vi "uc480_ImageSize.vi"() -> ()   [LabVIEW 2011]
uses:
  C:/Program Files/Thorlabs/Scientific Imaging/DCx Camera Support/Develop/DotNet/uc480DotNet.dll
  Develop/DotNet/uc480DotNet.dll
panel:
  out "Pos y":i32
  out "Pos x":i32
  out "AOI Height":i32
  out "AOI Width":i32
  in  "AOI - X Position":i32(slide)=33 min=0 max=0 step=2
  in  "AOI - Y Position":i32(slide)=33 min=0 max=0 step=2
  in  "AOI - Width":i32(slide)=16 min=16 max=1280 step=4 scale=16.0..1280.0
  in  "AOI - Height":i32(slide)=1 min=120 max=1024 step=2 scale=120.0..1024.0
  out "Image":picture
  in  "Camera ID":i32 min=0 max=255
  out "Serial Number":string
  out "Height":i32=8
  out "Width":i32=8
  out "Bits/Pixel":i32=8
  out "Error Out":errorcluster caption="error"
  in  "Exit Camera":bool
  in  "Init Camera":bool
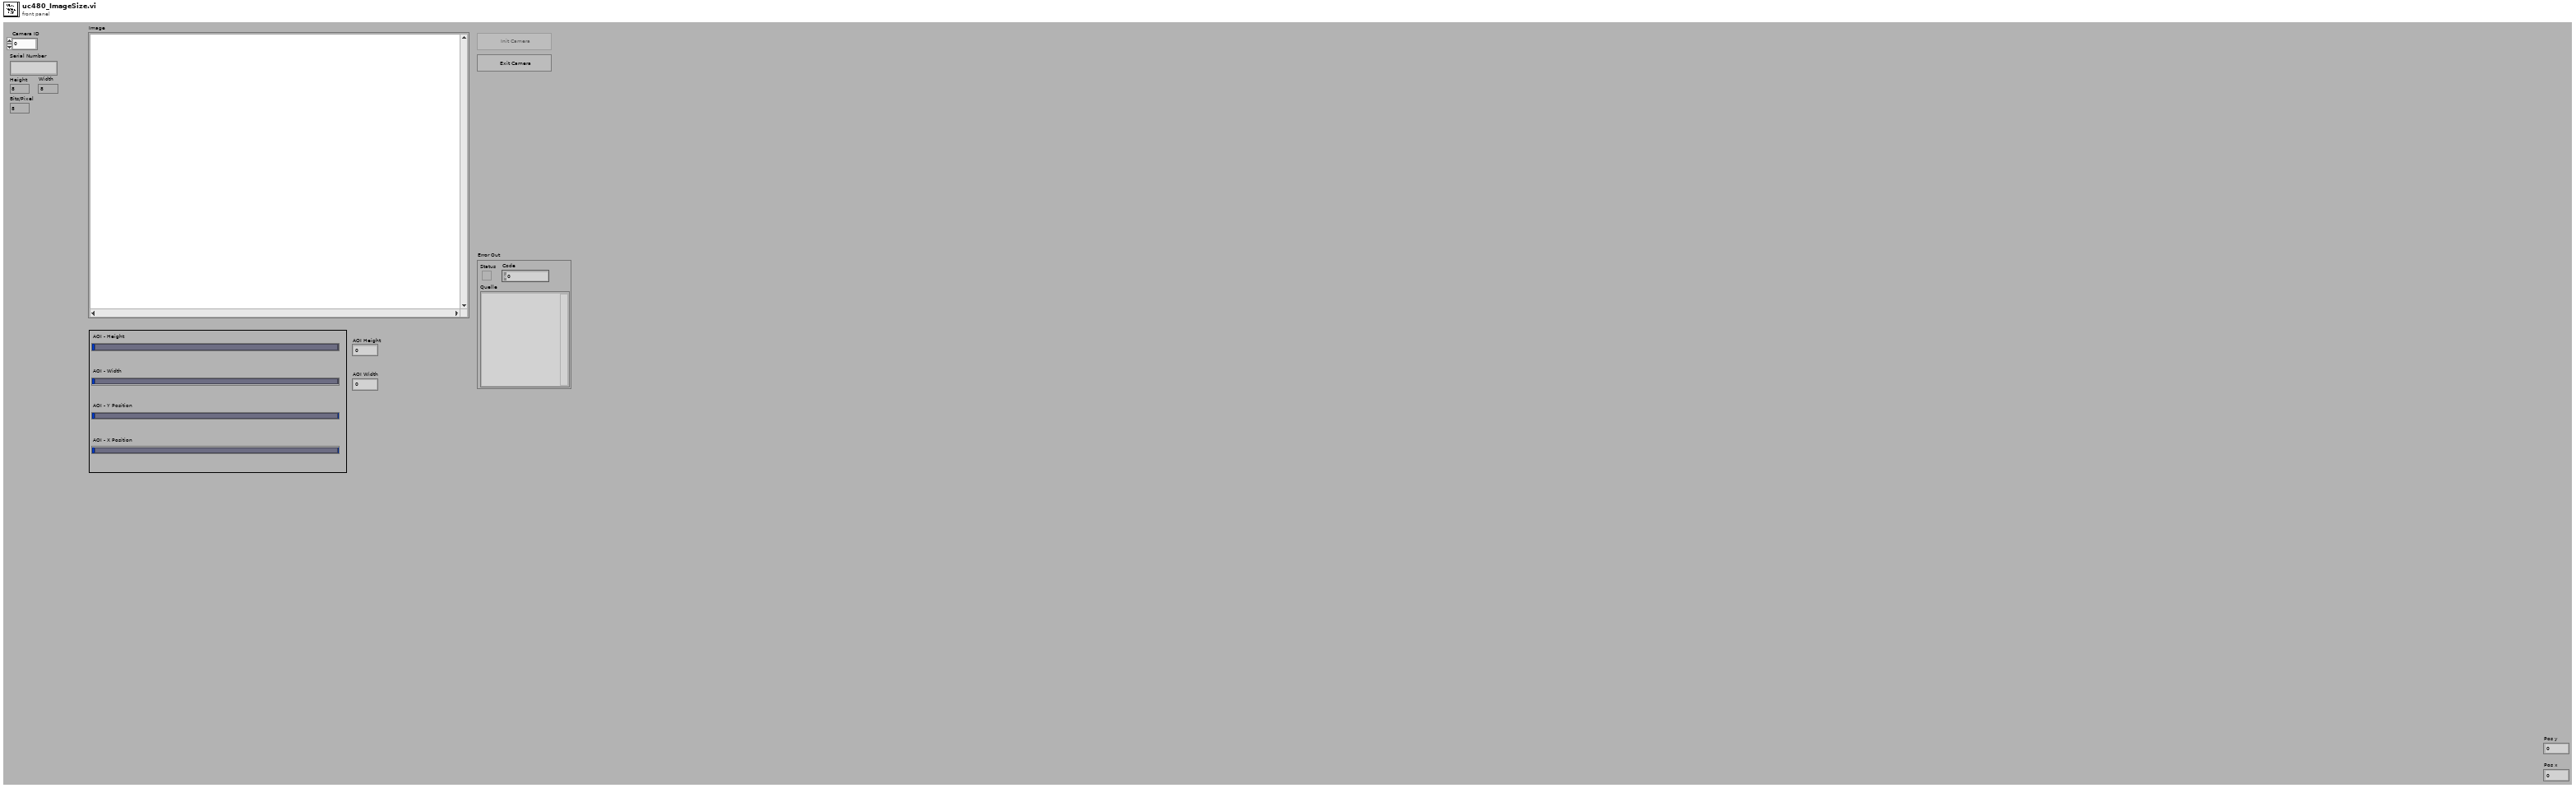
[diagram p1: front panel]
types:
  T1 = enum8{"Enabled", "Disabled", "Disabled and Grayed Out"}
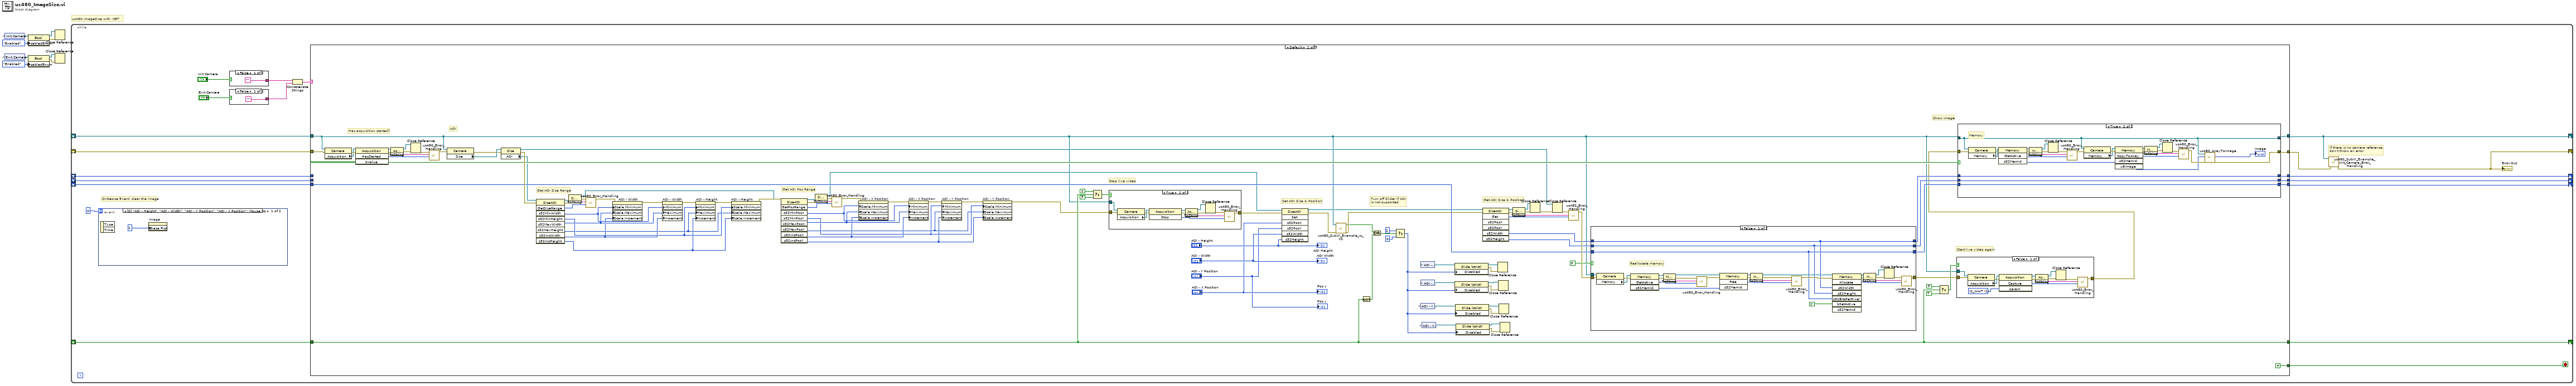
[diagram p0: block diagram]
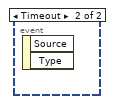
[diagram p2: hidden frame]
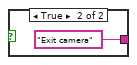
[diagram p3: hidden frame]
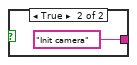
[diagram p4: hidden frame]
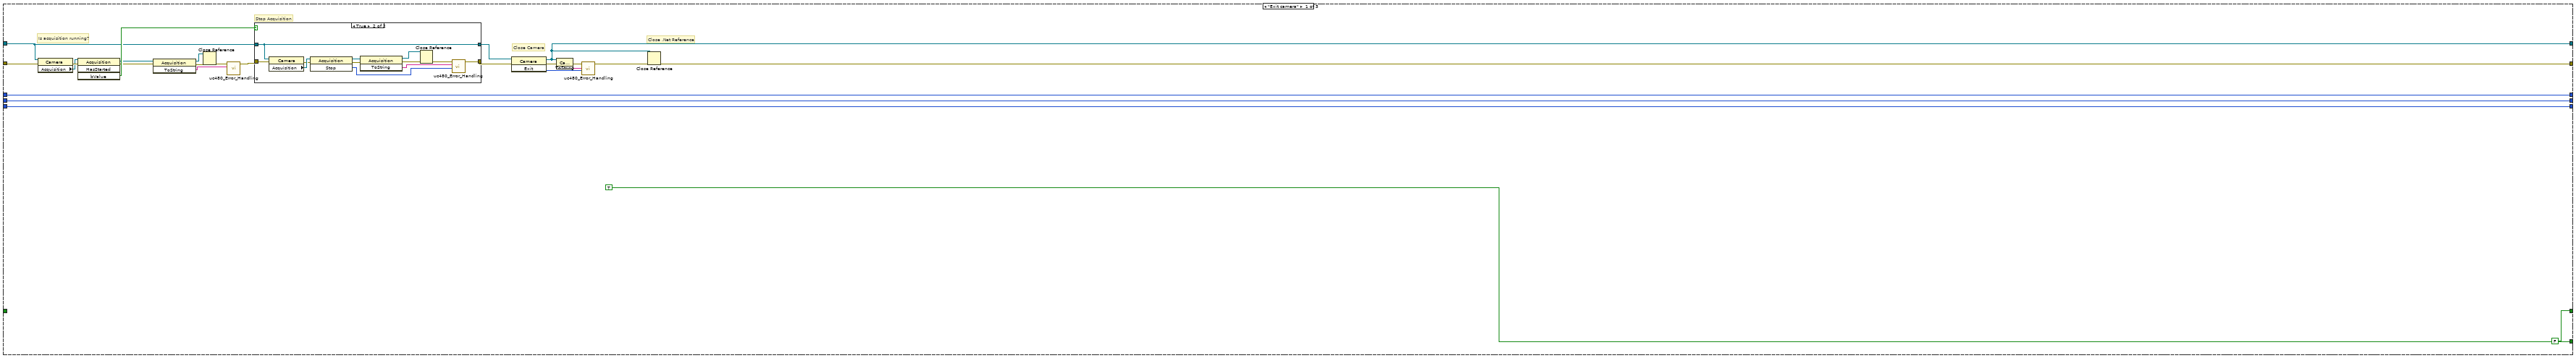
[diagram p5: hidden frame]
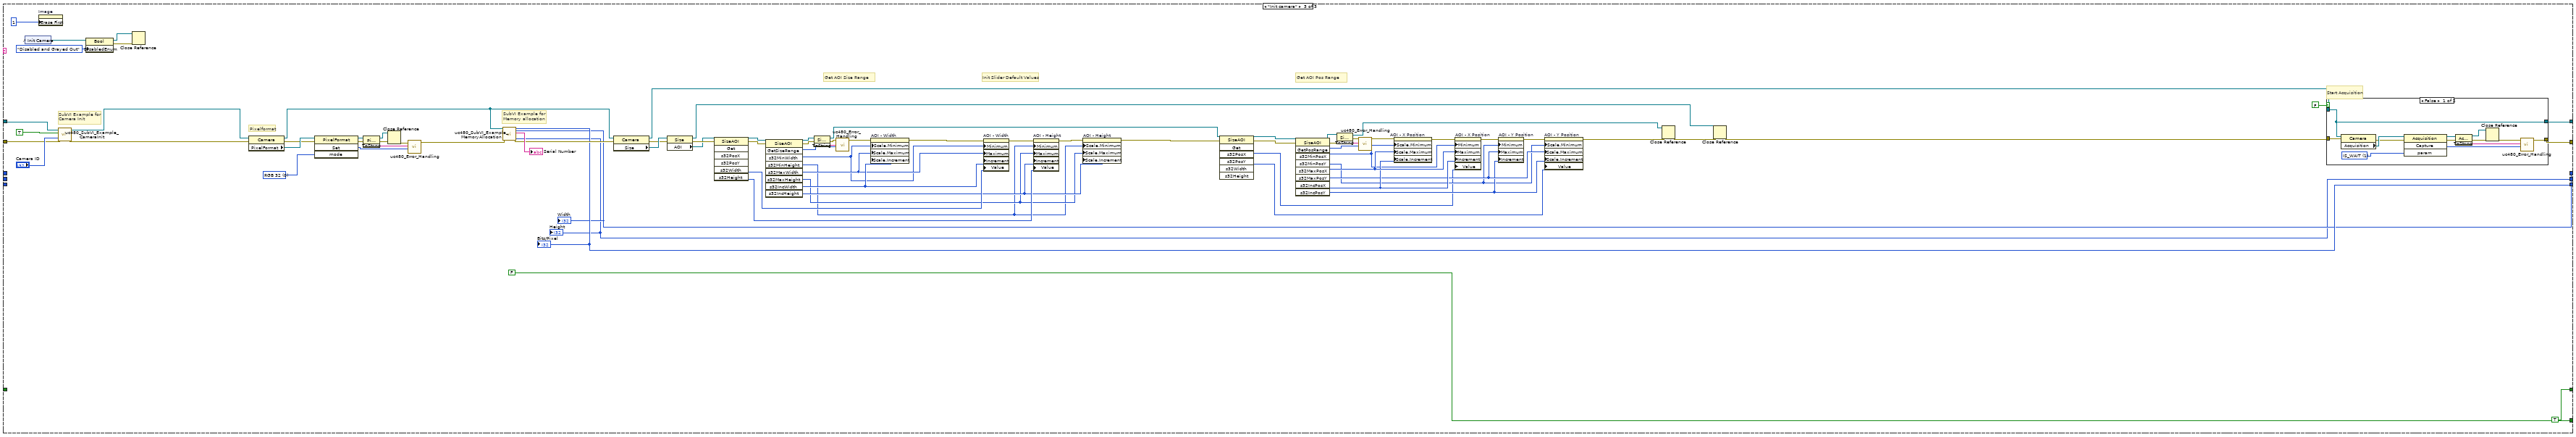
[diagram p11: hidden frame]
diagram:
  # "uc480 ImageSize with .NET"
  n1 = control-ref of="Init Camera"() -> (w5:refnum<vi>)
  n2 = control-ref of="Exit Camera"() -> (w7:refnum<vi>)
  n3 = property class="Bool"(reference=w5, "DisabledEnum"=T1."Enabled" ("Disabled")) -> (reference out=w3:refnum<vi>, error out=w4:errorcluster)  [unwired: 1 in]
  n4 = property class="Bool"(reference=w7, "DisabledEnum"=T1."Enabled" ("Disabled")) -> (reference out=w2:refnum<vi>, error out=w1:errorcluster)  [unwired: 1 in]
  n5 = Close Reference(reference=w2, error in (no error)=w1) -> ()  [unwired: 1 out]
  n6 = Close Reference(reference=w3, error in (no error)=w4) -> ()  [unwired: 1 out]
  n7 = while {
    shift-right: [w16] -> _
    shift-left: _ -> [w11]
    shift-right: [w15] -> _
    shift-left: _ -> [w9]
    shift-right: [w21] -> _
    shift-left: _ -> [w20]
    shift-right: [w23] -> _
    shift-left: _ -> [w19]
    shift-right: [w22] -> _
    shift-left: _ -> [w18]
    shift-right: [w13] -> _
    shift-left: _ -> [w12]
    stop <- w17 stop-if-true
    # "if there is no camera reference, \ndon't throw an error"
    # "OnResize Event, clear the image"
    n8 = event shown="[0] \"AOI - Height\", \"AOI - Width\", \"AOI - Y Position\", \"AOI - X Position\": Mouse Up" {
      selector: _ -> [_ _]
      dyn-events: _ -> [_ _]
      timeout: 0 -> [_ _]
      event "AOI - Height", "AOI - Width", "AOI - Y Position", "AOI - X Position": Mouse Up {
        n9 = event-data() -> ()  [unwired: 1 in, 2 out]
        n10 = property on="Image" class="Pict"("Erase First"=u8 1 ("Zuerst löschen")) -> ()  [unwired: 2 in, 2 out]
      }
      event Timeout {
        n11 = event-data() -> ()  [unwired: 1 in, 2 out]
      }
    }
    n12 = case shown="False" "Init Camera" {
      tunnel: ["" "Init camera"] -> w27
      frame False {
      }
      frame True {
      }
    }
    n13 = case shown="False" "Exit Camera" {
      tunnel: ["" "Exit camera"] -> w24
      frame False {
      }
      frame True {
      }
    }
    n14 = Concatenate Strings(w27, w24) -> (w26:string)
    n15 = case shown="Default" w26 {
      tunnel: w9 -> [w40 w98 w354]
      tunnel: w11 -> [w41 w99 w353]
      tunnel: [w52 w172 w324] -> w15
      tunnel: [w53 w171 w325] -> w10
      tunnel: [w51 w175 w314] -> w21
      tunnel: [w50 w174 w313] -> w23
      tunnel: [w49 w173 w315] -> w22
      tunnel: w20 -> [w51 _ _]
      tunnel: w19 -> [w50 _ _]
      tunnel: w18 -> [w49 w129 _]
      tunnel: [TRUE FALSE FALSE] -> w17
      tunnel: [FALSE w101 TRUE] -> w13
      tunnel: w12 -> [_ w101 _]
      frame "Exit camera" {
        # "Close .Net Reference"
        # "Is acquisition running?"
        # "Stop Acquisition"
        # "Close Camera"
        n16 = property class="Camera"(reference=w40, error in=w41) -> (error out=w48:errorcluster, "Acquisition"=w47:refnum<k24>)  [unwired: 1 out]
        n17 = invoke class="Acquisition" method="HasStarted"(reference=w47, error in=w48) -> (reference out=w42:refnum<k24>, error out=w44:errorcluster, "bValue"=w46:bool)  [unwired: 2 in, 1 out]
        n18 = invoke class="Acquisition" method="ToString"(reference=w42, error in=w44) -> (reference out=w34:refnum<k24>, error out=w36:errorcluster, "ToString"=w43:string)  [unwired: 1 in]
        n19 = Close Reference(reference=w34, error in (no error)=w36) -> (error out=w35:errorcluster)
        n20 = call "uc480_Error_Handling.vi"("Error String"=w43, "Error In"=w35) -> ("Error Out"=w45:errorcluster)  [unwired: 9 in]
        n21 = case shown="True" w46 {
          tunnel: [w61 w72] -> w38
          tunnel: w45 -> [w61 w73]
          tunnel: w40 -> [w60 w65]
          tunnel: [w60 w65] -> w39
          frame False {
          }
          frame True {
            n22 = property class="Camera"(reference=w65, error in=w73) -> (error out=w69:errorcluster, "Acquisition"=w70:refnum<k24>)  [unwired: 1 out]
            n23 = invoke class="Acquisition" method="Stop"(reference=w70, error in=w69) -> (reference out=w67:refnum<k24>, error out=w68:errorcluster, "Stop"=w66:i32)  [unwired: 1 in]
            n24 = invoke class="Acquisition" method="ToString"(reference=w67, error in=w68) -> (reference out=w62:refnum<k24>, error out=w64:errorcluster, "ToString"=w71:string)  [unwired: 1 in]
            n25 = Close Reference(reference=w62, error in (no error)=w64) -> (error out=w63:errorcluster)
            n26 = call "uc480_Error_Handling.vi"("Error Code"=w66, "Error String"=w71, "Error In"=w63) -> ("Error Out"=w72:errorcluster)  [unwired: 8 in]
          }
        }
        n27 = invoke class="Camera" method="Exit"(reference=w39, error in=w38) -> (reference out=w52:refnum<k24>, error out=w56:errorcluster, "Exit"=w55:i32)  [unwired: 1 in]
        n28 = invoke class="Camera" method="ToString"(reference=w52, error in=w56) -> (error out=w57:errorcluster, "ToString"=w58:string)  [unwired: 1 in, 1 out]
        n29 = call "uc480_Error_Handling.vi"("Error Code"=w55, "Error String"=w58, "Error In"=w57) -> ("Error Out"=w54:errorcluster)  [unwired: 8 in]
        n30 = Close Reference ("Close Referenz")(reference=w52, error in (no error)=w54) -> (error out=w53:errorcluster)
      }
      frame Default {
        # "Turn off Slider if AOI\nis not supported"
        # "Start live video again"
        # "Stop live video"
        # "Get AOI Size & Position"
        # "Set AOI Size & Position"
        # "Get AOI Pos Range"
        # "Get AOI Size Range"
        # "AOI"
        # "Has acquisition started?"
        # "Show Image"
        n31 = property class="Camera"(reference=w98, error in=w99) -> (error out=w181:errorcluster, "Acquisition"=w180:refnum<k24>)  [unwired: 1 out]
        n32 = invoke class="Acquisition" method="HasStarted"(reference=w180, error in=w181) -> (reference out=w178:refnum<k24>, error out=w177:errorcluster, "HasStarted"=w176:i32, "bValue"=w125:bool)  [unwired: 2 in]
        n33 = invoke class="Acquisition" method="ToString"(reference=w178, error in=w177) -> (reference out=w92:refnum<k24>, error out=w94:errorcluster, "ToString"=w179:string)  [unwired: 1 in]
        n34 = Close Reference(reference=w92, error in (no error)=w94) -> (error out=w93:errorcluster)
        n35 = call "uc480_Error_Handling.vi"("Error Code"=w176, "Error String"=w179, "Error In"=w93) -> ("Error Out"=w170:errorcluster)  [unwired: 8 in]
        n36 = property class="Camera"(reference=w98, error in=w170) -> (error out=w168:errorcluster, "Size"=w169:refnum<k24>)  [unwired: 1 out]
        n37 = property class="Size"(reference=w169, error in=w168) -> (reference out=w83:refnum<k24>, error out=w167:errorcluster, "AOI"=w86:refnum<k24>)
        n38 = invoke class="SizeAOI" method="GetSizeRange"(reference=w86, error in=w167) -> (reference out=w162:refnum<k24>, error out=w163:errorcluster, "GetSizeRange"=w164:i32, "s32MinWidth"=w156:i32, "s32MinHeight"=w153:i32, "s32MaxWidth"=w155:i32, "s32MaxHeight"=w152:i32, "s32IncWidth"=w154:i32, "s32IncHeight"=w151:i32)  [unwired: 7 in]
        n39 = invoke class="SizeAOI" method="ToString"(reference=w162, error in=w163) -> (reference out=w91:refnum<k24>, error out=w166:errorcluster, "ToString"=w165:string)  [unwired: 1 in]
        n40 = call "uc480_Error_Handling.vi"("Error Code"=w164, "Error String"=w165, "Error In"=w166) -> ("Error Out"=w161:errorcluster)  [unwired: 8 in]
        n41 = property on="AOI - Width" class="Slide (strict)"(error in=w161, "Scale.Minimum"=w156, "Scale.Maximum"=w155, "Scale.Increment"=w154) -> (error out=w150:errorcluster)  [unwired: 1 in, 1 out]
        n42 = property on="AOI - Width" class="Slide (strict)"(error in=w150, "Minimum"=w156, "Maximum"=w155, "Increment"=w154) -> (error out=w120:errorcluster)  [unwired: 1 in, 1 out]
        n43 = property on="AOI - Height" class="Slide (strict)"(error in=w120, "Minimum"=w153, "Maximum"=w152, "Increment"=w151) -> (error out=w149:errorcluster)  [unwired: 1 in, 1 out]
        n44 = property on="AOI - Height" class="Slide (strict)"(error in=w149, "Scale.Minimum"=w153, "Scale.Maximum"=w152, "Scale.Increment"=w151) -> (error out=w133:errorcluster)  [unwired: 1 in, 1 out]
        n45 = invoke class="SizeAOI" method="GetPosRange"(reference=w91, error in=w133) -> (reference out=w144:refnum<k24>, error out=w145:errorcluster, "GetPosRange"=w146:i32, "s32MinPosX"=w142:i32, "s32MinPosY"=w138:i32, "s32MaxPosX"=w141:i32, "s32MaxPosY"=w137:i32, "s32IncPosX"=w140:i32, "s32IncPosY"=w136:i32)  [unwired: 7 in]
        n46 = invoke class="SizeAOI" method="ToString"(reference=w144, error in=w145) -> (reference out=w85:refnum<k24>, error out=w148:errorcluster, "ToString"=w147:string)  [unwired: 1 in]
        n47 = call "uc480_Error_Handling.vi"("Error Code"=w146, "Error String"=w147, "Error In"=w148) -> ("Error Out"=w143:errorcluster)  [unwired: 8 in]
        n48 = property on="AOI - X Position" class="Slide (strict)"(error in=w143, "Scale.Minimum"=w142, "Scale.Maximum"=w141, "Scale.Increment"=w140) -> (error out=w135:errorcluster)  [unwired: 1 in, 1 out]
        n49 = property on="AOI - X Position" class="Slide (strict)"(error in=w135, "Minimum"=w142, "Maximum"=w141, "Increment"=w140) -> (error out=w139:errorcluster)  [unwired: 1 in, 1 out]
        n50 = property on="AOI - Y Position" class="Slide (strict)"(error in=w139, "Minimum"=w138, "Maximum"=w137, "Increment"=w136) -> (error out=w134:errorcluster)  [unwired: 1 in, 1 out]
        n51 = property on="AOI - Y Position" class="Slide (strict)"(error in=w134, "Scale.Minimum"=w138, "Scale.Maximum"=w137, "Scale.Increment"=w136) -> (error out=w87:errorcluster)  [unwired: 1 in, 1 out]
        n52 = Select(t=TRUE, s=w101, f=FALSE) -> (s? t:f=w110:bool)
        n53 = case shown="True" w110 {
          tunnel: [w183 w194] -> w124
          tunnel: w87 -> [w183 w195]
          tunnel: w98 -> [_ w187]
          frame False {
          }
          frame True {
            n54 = property class="Camera"(reference=w187, error in=w195) -> (error out=w191:errorcluster, "Acquisition"=w192:refnum<k24>)  [unwired: 1 out]
            n55 = invoke class="Acquisition" method="Stop"(reference=w192, error in=w191) -> (reference out=w189:refnum<k24>, error out=w190:errorcluster, "Stop"=w188:i32)  [unwired: 1 in]
            n56 = invoke class="Acquisition" method="ToString"(reference=w189, error in=w190) -> (reference out=w184:refnum<k24>, error out=w186:errorcluster, "ToString"=w193:string)  [unwired: 1 in]
            n57 = Close Reference(reference=w184, error in (no error)=w186) -> (error out=w185:errorcluster)
            n58 = call "uc480_Error_Handling.vi"("Error Code"=w188, "Error String"=w193, "Error In"=w185) -> ("Error Out"=w194:errorcluster)  [unwired: 8 in]
          }
        }
        n59 = invoke class="SizeAOI" method="Set"(reference=w85, error in=w124, "s32PosX"="AOI - X Position", "s32PosY"="AOI - Y Position", "s32Width"="AOI - Width", "s32Height"="AOI - Height") -> (reference out=w90:refnum<k24>, error out=w97:errorcluster)  [unwired: 1 in, 5 out]
        n60 = call "uc480_SubVI_Example_Is_XS.vi"("Error In"=w97, ".NET (Reference)"=w98) -> ("Error Out"=w96:errorcluster, "IsXS"=w95:bool)  [unwired: 7 in, 1 out]
        n61 = Not(x=w101) -> (.not. x?=w100:bool)
        n62 = Or(x=w95, y=w100) -> (x .or. y?=w102:bool)
        n63 = Select(t=2 ("y"), s=w102, f=0 ("y")) -> (s? t:f=w103:i32)
        n64 = control-ref of="AOI - Y Position"() -> (w108:refnum<vi>)
        n65 = control-ref of="AOI - Height"() -> (w106:refnum<vi>)
        n66 = control-ref of="AOI - Width"() -> (w107:refnum<vi>)
        n67 = control-ref of="AOI - X Position"() -> (w109:refnum<vi>)
        n68 = property class="Slide (strict)"(reference=w106, "Disabled"=w103) -> (reference out=w74:refnum<vi>, error out=w81:errorcluster)  [unwired: 1 in]
        n69 = property class="Slide (strict)"(reference=w107, "Disabled"=w103) -> (reference out=w76:refnum<vi>, error out=w75:errorcluster)  [unwired: 1 in]
        n70 = property class="Slide (strict)"(reference=w108, "Disabled"=w103) -> (reference out=w78:refnum<vi>, error out=w77:errorcluster)  [unwired: 1 in]
        n71 = property class="Slide (strict)"(reference=w109, "Disabled"=w103) -> (reference out=w79:refnum<vi>, error out=w80:errorcluster)  [unwired: 1 in]
        n72 = invoke class="SizeAOI" method="Get"(reference=w90, error in=w96) -> (reference out=w159:refnum<k24>, error out=w158:errorcluster, "Get"=w157:i32, "s32Width"=w131:i32, "s32Height"=w130:i32)  [unwired: 5 in, 2 out]
        n73 = Close Reference(reference=w74, error in (no error)=w81) -> ()  [unwired: 1 out]
        n74 = Close Reference(reference=w76, error in (no error)=w75) -> ()  [unwired: 1 out]
        n75 = Close Reference(reference=w78, error in (no error)=w77) -> ()  [unwired: 1 out]
        n76 = Close Reference(reference=w79, error in (no error)=w80) -> ()  [unwired: 1 out]
        n77 = invoke class="SizeAOI" method="ToString"(reference=w159, error in=w158) -> (reference out=w88:refnum<k24>, error out=w89:errorcluster, "ToString"=w160:string)  [unwired: 1 in]
        n78 = Close Reference(reference=w88, error in (no error)=w89) -> (error out=w84:errorcluster)
        n79 = Close Reference(reference=w83, error in (no error)=w84) -> (error out=w82:errorcluster)
        n80 = call "uc480_Error_Handling.vi"("Error Code"=w157, "Error String"=w160, "Error In"=w82) -> ("Error Out"=w132:errorcluster)  [unwired: 8 in]
        n81 = case shown="False" FALSE {
          tunnel: w132 -> [w223 w241]
          tunnel: w131 -> [w219 w244]
          tunnel: w130 -> [w220 w243]
          tunnel: w129 -> [w221 w242]
          tunnel: [w222 w241] -> w123
          tunnel: [w221 w242] -> w128
          tunnel: [w220 w243] -> w127
          tunnel: [w219 w244] -> w126
          tunnel: w98 -> [w218 _]
          frame False {
            # "Reallocate memory"
            n82 = property class="Camera"(reference=w218, error in=w223) -> (error out=w225:errorcluster, "Memory"=w217:refnum<k24>)  [unwired: 1 out]
            n83 = invoke class="Memory" method="GetActive"(reference=w217, error in=w225) -> (reference out=w230:refnum<k24>, error out=w229:errorcluster, "GetActive"=w228:i32, "s32MemId"=w227:i32)  [unwired: 2 in]
            n84 = invoke class="Memory" method="ToString"(reference=w230, error in=w229) -> (reference out=w216:refnum<k24>, error out=w215:errorcluster, "ToString"=w231:string)  [unwired: 1 in]
            n85 = call "uc480_Error_Handling.vi"("Error Code"=w228, "Error String"=w231, "Error In"=w215) -> ("Error Out"=w226:errorcluster)  [unwired: 8 in]
            n86 = invoke class="Memory" method="Free"(reference=w216, error in=w226, "s32MemId"=w227) -> (reference out=w234:refnum<k24>, error out=w233:errorcluster, "Free"=w232:i32)  [unwired: 1 in, 1 out]
            n87 = invoke class="Memory" method="ToString"(reference=w234, error in=w233) -> (reference out=w213:refnum<k24>, error out=w214:errorcluster, "ToString"=w235:string)  [unwired: 1 in]
            n88 = call "uc480_Error_Handling.vi"("Error Code"=w232, "Error String"=w235, "Error In"=w214) -> ("Error Out"=w224:errorcluster)  [unwired: 8 in]
            n89 = invoke class="Memory" method="Allocate"(reference=w213, error in=w224, "s32Width"=w219, "s32Height"=w220, "s32BitsPerPixel"=w221, "bSetActive"=TRUE) -> (reference out=w239:refnum<k24>, error out=w238:errorcluster, "Allocate"=w237:i32)  [unwired: 2 in, 5 out]
            n90 = invoke class="Memory" method="ToString"(reference=w239, error in=w238) -> (reference out=w210:refnum<k24>, error out=w212:errorcluster, "ToString"=w240:string)  [unwired: 1 in]
            n91 = Close Reference(reference=w210, error in (no error)=w212) -> (error out=w211:errorcluster)
            n92 = call "uc480_Error_Handling.vi"("Error Code"=w237, "Error String"=w240, "Error In"=w211) -> ("Error Out"=w222:errorcluster)  [unwired: 8 in]
          }
          frame True {
          }
        }
        n93 = Select(t=FALSE, s=w101, f=TRUE) -> (s? t:f=w113:bool)
        n94 = case shown="False" w113 {
          tunnel: [w201 w209] -> w122
          tunnel: w123 -> [w206 w209]
          tunnel: w98 -> [w205 _]
          frame False {
            w199 = 1 items=["IS_DONT_WAIT", "IS_WAIT"] ("Wait")
            n95 = property class="Camera"(reference=w205, error in=w206) -> (error out=w207:errorcluster, "Acquisition"=w208:refnum<k24>)  [unwired: 1 out]
            n96 = invoke class="Acquisition" method="Capture"(reference=w208, error in=w207, "param"=w199) -> (reference out=w202:refnum<k24>, error out=w203:errorcluster, "Capture"=w200:i32)  [unwired: 1 in, 1 out]
            n97 = invoke class="Acquisition" method="ToString"(reference=w202, error in=w203) -> (reference out=w196:refnum<k24>, error out=w198:errorcluster, "ToString"=w204:string)  [unwired: 1 in]
            n98 = Close Reference(reference=w196, error in (no error)=w198) -> (error out=w197:errorcluster)
            n99 = call "uc480_Error_Handling.vi"("Error Code"=w200, "Error String"=w204, "Error In"=w197) -> ("Error Out"=w201:errorcluster)  [unwired: 8 in]
          }
          frame True {
          }
        }
        n100 = case shown="True" w125 {
          tunnel: [w249 w264] -> w171
          tunnel: w122 -> [w249 w260]
          tunnel: w98 -> [w248 w256]
          tunnel: [w248 w256] -> w172
          tunnel: w126 -> [w247 w263]
          tunnel: w127 -> [w246 w262]
          tunnel: w128 -> [w245 w261]
          tunnel: [w247 w263] -> w175
          tunnel: [w246 w262] -> w174
          tunnel: [w245 w261] -> w173
          frame False {
          }
          frame True {
            # "Memory"
            n101 = property class="Camera"(reference=w256, error in=w260) -> (error out=w266:errorcluster, "Memory"=w267:refnum<k24>)  [unwired: 1 out]
            n102 = invoke class="Memory" method="GetActive"(reference=w267, error in=w266) -> (reference out=w272:refnum<k24>, error out=w271:errorcluster, "GetActive"=w273:i32, "s32MemId"=w265:i32)  [unwired: 2 in]
            n103 = invoke class="Memory" method="ToString"(reference=w272, error in=w271) -> (reference out=w253:refnum<k24>, error out=w255:errorcluster, "ToString"=w270:string)  [unwired: 1 in]
            n104 = Close Reference(reference=w253, error in (no error)=w255) -> (error out=w254:errorcluster)
            n105 = call "uc480_Error_Handling.vi"("Error Code"=w273, "Error String"=w270, "Error In"=w254) -> ("Error Out"=w274:errorcluster)  [unwired: 8 in]
            n106 = property class="Camera"(reference=w256, error in=w274) -> (error out=w269:errorcluster, "Memory"=w268:refnum<k24>)  [unwired: 1 out]
            n107 = invoke class="Memory" method="CopyToArray"(reference=w268, error in=w269, "s32MemId"=w265) -> (reference out=w276:refnum<k24>, error out=w277:errorcluster, "CopyToArray"=w278:i32, "u8Image"=w257:u8[])  [unwired: 2 in, 1 out]
            n108 = invoke class="Memory" method="ToString"(reference=w276, error in=w277) -> (reference out=w250:refnum<k24>, error out=w252:errorcluster, "ToString"=w275:string)  [unwired: 1 in]
            n109 = Close Reference(reference=w250, error in (no error)=w252) -> (error out=w251:errorcluster)
            n110 = call "uc480_Error_Handling.vi"("Error Code"=w278, "Error String"=w275, "Error In"=w251) -> ("Error Out"=w258:errorcluster)  [unwired: 8 in]
            n111 = call "uc480_ArrayToImage.vi"("Error In"=w258, "InArray"=w257, ".NET (Reference)"=w256) -> ("Error Out"=w264:errorcluster, "Image"=→"Image":picture)  [unwired: 7 in]
          }
        }
        "AOI Width" <- "AOI - Width"
        "AOI Height" <- "AOI - Height"
        "Pos x" <- "AOI - X Position"
        "Pos y" <- "AOI - Y Position"
      }
      frame "Init camera" {
        w361 = 0 items=["RGB 32"=0, "RGB 24"=1, "Y8 Monochrom"=6] ("Mode")
        # "Start Acquisition"
        # "Init Slider Default Values"
        # "Get AOI Pos Range"
        # "Get AOI Size Range"
        # "SubVI Example for \nMemory allocation"
        # "SubVI Example for \nCamera Init"
        # "Pixelformat"
        n112 = control-ref of="Init Camera"() -> (w317:refnum<vi>)
        n113 = property on="Image" class="Pict"("Erase First"=u8 1 ("Zuerst löschen")) -> ()  [unwired: 2 in, 2 out]
        n114 = call "uc480_SubVI_Example_CameraInit.vi"("Error In"=w353, "Camera ID"="Camera ID", "Init Camera Flag"=TRUE, ".NET (Reference)"=w354) -> ("Error Out"=w320:errorcluster, ".NET (Reference)"=w282:refnum<k24>)  [unwired: 6 in]
        n115 = property class="Bool"(reference=w317, "DisabledEnum"=T1."Disabled and Grayed Out" ("Disabled")) -> (reference out=w280:refnum<vi>, error out=w279:errorcluster)  [unwired: 1 in]
        n116 = Close Reference(reference=w280, error in (no error)=w279) -> ()  [unwired: 1 out]
        n117 = property class="Camera"(reference=w282, error in=w320) -> (reference out=w281:refnum<k24>, error out=w359:errorcluster, "PixelFormat"=w360:refnum<k24>)
        n118 = invoke class="PixelFormat" method="Set"(reference=w360, error in=w359, "mode"=w361) -> (reference out=w357:refnum<k24>, error out=w350:errorcluster, "Set"=w356:i32)  [unwired: 1 in, 1 out]
        n119 = invoke class="PixelFormat" method="ToString"(reference=w357, error in=w350) -> (reference out=w292:refnum<k24>, error out=w294:errorcluster, "ToString"=w358:string)  [unwired: 1 in]
        n120 = Close Reference(reference=w292, error in (no error)=w294) -> (error out=w293:errorcluster)
        n121 = call "uc480_Error_Handling.vi"("Error Code"=w356, "Error String"=w358, "Error In"=w293) -> ("Error Out"=w319:errorcluster)  [unwired: 8 in]
        n122 = call "uc480_SubVI_Example_MemoryAllocation.vi"(".NET (Reference)"=w281, "Error In"=w319) -> ("Bits/Pixel 2"=w315:i32, "Width"=w314:i32, "Serial Number"=→"Serial Number":string, "Height"=w313:i32, "Error Out"=w341:errorcluster)  [unwired: 13 in]
        "Bits/Pixel" <- w315
        "Width" <- w314
        "Height" <- w313
        n123 = property class="Camera"(reference=w281, error in=w341) -> (reference out=w291:refnum<k24>, error out=w321:errorcluster, "Size"=w322:refnum<k24>)
        n124 = property class="Size"(reference=w322, error in=w321) -> (reference out=w287:refnum<k24>, error out=w310:errorcluster, "AOI"=w295:refnum<k24>)
        n125 = invoke class="SizeAOI" method="Get"(reference=w295, error in=w310) -> (reference out=w311:refnum<k24>, error out=w309:errorcluster, "s32Width"=w303:i32, "s32Height"=w302:i32)  [unwired: 5 in, 3 out]
        n126 = invoke class="SizeAOI" method="GetSizeRange"(reference=w311, error in=w309) -> (reference out=w345:refnum<k24>, error out=w346:errorcluster, "GetSizeRange"=w308:i32, "s32MinWidth"=w304:i32, "s32MinHeight"=w299:i32, "s32MaxWidth"=w305:i32, "s32MaxHeight"=w300:i32, "s32IncWidth"=w306:i32, "s32IncHeight"=w301:i32)  [unwired: 7 in]
        n127 = invoke class="SizeAOI" method="ToString"(reference=w345, error in=w346) -> (reference out=w283:refnum<k24>, error out=w348:errorcluster, "ToString"=w347:string)  [unwired: 1 in]
        n128 = call "uc480_Error_Handling.vi"("Error Code"=w308, "Error String"=w347, "Error In"=w348) -> ("Error Out"=w307:errorcluster)  [unwired: 8 in]
        n129 = property on="AOI - Width" class="Slide (strict)"(error in=w307, "Scale.Minimum"=w304, "Scale.Maximum"=w305, "Scale.Increment"=w306) -> (error out=w343:errorcluster)  [unwired: 1 in, 1 out]
        n130 = property on="AOI - Width" class="Slide (strict)"(error in=w343, "Minimum"=w304, "Maximum"=w305, "Increment"=w306, "Value"=w303) -> (error out=w344:errorcluster)  [unwired: 1 in, 1 out]
        n131 = property on="AOI - Height" class="Slide (strict)"(error in=w344, "Minimum"=w299, "Maximum"=w300, "Increment"=w301, "Value"=w302) -> (error out=w342:errorcluster)  [unwired: 1 in, 1 out]
        n132 = property on="AOI - Height" class="Slide (strict)"(error in=w342, "Scale.Minimum"=w299, "Scale.Maximum"=w300, "Scale.Increment"=w301) -> (error out=w284:errorcluster)  [unwired: 1 in, 1 out]
        n133 = invoke class="SizeAOI" method="Get"(reference=w283, error in=w284) -> (reference out=w285:refnum<k24>, error out=w298:errorcluster, "s32PosX"=w297:i32, "s32PosY"=w296:i32)  [unwired: 5 in, 3 out]
        n134 = invoke class="SizeAOI" method="GetPosRange"(reference=w285, error in=w298) -> (reference out=w336:refnum<k24>, error out=w337:errorcluster, "GetPosRange"=w338:i32, "s32MinPosX"=w312:i32, "s32MinPosY"=w327:i32, "s32MaxPosX"=w334:i32, "s32MaxPosY"=w331:i32, "s32IncPosX"=w333:i32, "s32IncPosY"=w330:i32)  [unwired: 7 in]
        n135 = invoke class="SizeAOI" method="ToString"(reference=w336, error in=w337) -> (reference out=w289:refnum<k24>, error out=w340:errorcluster, "ToString"=w339:string)  [unwired: 1 in]
        n136 = call "uc480_Error_Handling.vi"("Error Code"=w338, "Error String"=w339, "Error In"=w340) -> ("Error Out"=w335:errorcluster)  [unwired: 8 in]
        n137 = property on="AOI - X Position" class="Slide (strict)"(error in=w335, "Scale.Minimum"=w312, "Scale.Maximum"=w334, "Scale.Increment"=w333) -> (error out=w329:errorcluster)  [unwired: 1 in, 1 out]
        n138 = property on="AOI - X Position" class="Slide (strict)"(error in=w329, "Minimum"=w312, "Maximum"=w334, "Increment"=w333, "Value"=w297) -> (error out=w332:errorcluster)  [unwired: 1 in, 1 out]
        n139 = property on="AOI - Y Position" class="Slide (strict)"(error in=w332, "Minimum"=w327, "Maximum"=w331, "Increment"=w330) -> (error out=w328:errorcluster)  [unwired: 1 in, 1 out]
        n140 = property on="AOI - Y Position" class="Slide (strict)"(error in=w328, "Scale.Minimum"=w327, "Scale.Maximum"=w331, "Scale.Increment"=w330, "Value"=w296) -> (error out=w290:errorcluster)  [unwired: 1 in, 1 out]
        n141 = Close Reference(reference=w289, error in (no error)=w290) -> (error out=w288:errorcluster)
        n142 = Close Reference(reference=w287, error in (no error)=w288) -> (error out=w286:errorcluster)
        n143 = case shown="False" FALSE {
          tunnel: [w367 w376] -> w325
          tunnel: w286 -> [w372 w376]
          tunnel: w291 -> [w371 w375]
          tunnel: [w371 w375] -> w324
          frame False {
            w365 = 1 items=["IS_DONT_WAIT", "IS_WAIT"] ("Wait")
            n144 = property class="Camera"(reference=w371, error in=w372) -> (error out=w373:errorcluster, "Acquisition"=w374:refnum<k24>)  [unwired: 1 out]
            n145 = invoke class="Acquisition" method="Capture"(reference=w374, error in=w373, "param"=w365) -> (reference out=w368:refnum<k24>, error out=w369:errorcluster, "Capture"=w366:i32)  [unwired: 1 in, 1 out]
            n146 = invoke class="Acquisition" method="ToString"(reference=w368, error in=w369) -> (reference out=w362:refnum<k24>, error out=w364:errorcluster, "ToString"=w370:string)  [unwired: 1 in]
            n147 = Close Reference(reference=w362, error in (no error)=w364) -> (error out=w363:errorcluster)
            n148 = call "uc480_Error_Handling.vi"("Error Code"=w366, "Error String"=w370, "Error In"=w363) -> ("Error Out"=w367:errorcluster)  [unwired: 8 in]
          }
          frame True {
          }
        }
      }
    }
    n149 = call "uc480_SubVI_Example_Init_Camera_Error_Handling.vi"("Error In"=w10, ".NET (Reference)"=w15) -> ("Error Out"=w16:errorcluster)  [unwired: 9 in]
    "Error Out" <- w16
  }
